vi "PICRv1.vi"() -> ()   [LabVIEW 2013]
uses:
  <vilib>/MakerHub/LINX/Public/Sensors/Accelerometer/MPU60X0/DeviceAddresses.ctl
  <vilib>/MakerHub/LINX/Public/Sensors/Accelerometer/MPU60X0/AccelFullScaleRanges.ctl
  <vilib>/MakerHub/LINX/Public/Sensors/Accelerometer/MPU60X0/GyroFullScaleRanges.ctl
  <vilib>/vision/Avi.llb/IMAQ AVI2 Refnum.ctl
  <vilib>/MakerHub/LINX/Public/Peripherals/Digital/Digital Write 1 Chan.vi
  <vilib>/MakerHub/LINX/Public/Peripherals/Digital/Digital Write N Chans.vi
  <vilib>/MakerHub/LINX/Private/Local IO/LinxDigitalWrite.vi
  <vilib>/MakerHub/LINX/Public/Utilities/Check Channel.vi
  <vilib>/MakerHub/LINX/Public/Utilities/Open Serial.vi
  <vilib>/MakerHub/LINX/Private/Utilties/Generate Error.vi
  <vilib>/picture/3D Picture Control/Object/Create Object (name).vi
  <vilib>/MakerHub/LINX/LMH-LINX.lvlib
  <vilib>/MakerHub/LINX/Public/Sensors/Accelerometer/MPU60X0/MPU60X0.lvlib
  <vilib>/picture/3D Picture Control/NI_3D Picture Control.lvlib
  <vilib>/vision/driver/NI_Vision_Acquisition_Software.lvlib
panel:
  out "Pressure":dbl
  in  "Stop":bool
  out "Image":T1(plugin-control)
  in  "Record":bool
  in  "AVI File Path":path=path "C:/Users/Deyaa/Desktop/op1.avi"
  in  "Motors":bool
  in  "Brush":bool
  in  "Stop/Start":bool
  out "Acceleration":T2(graph)
  in  "stop":bool
  out "Start/ Stop":bool
  out "Brush":bool
  out "Motors":bool
  in  "Slide":dbl(slide) scale=1.0..100.0
  out "3D Picture":refnum<vi>(3d-picture)
  out "Gyroscope":T2(graph)
  out "Temperature (°C)":dbl
  out "Acceleration  (dps)":T2
  in  "Stop":bool
  out "Gyro (g)":T2
  # "Gyroscope Simulation"
  # "Camera"
  # "IMU"
  # "Motion"
  # "Sinai University - Department Of Mechatronics\nGraduation Project 2017\nUnder Supervision Of Prof. Saber Abdrabbo\nDeyaa Muhammad"
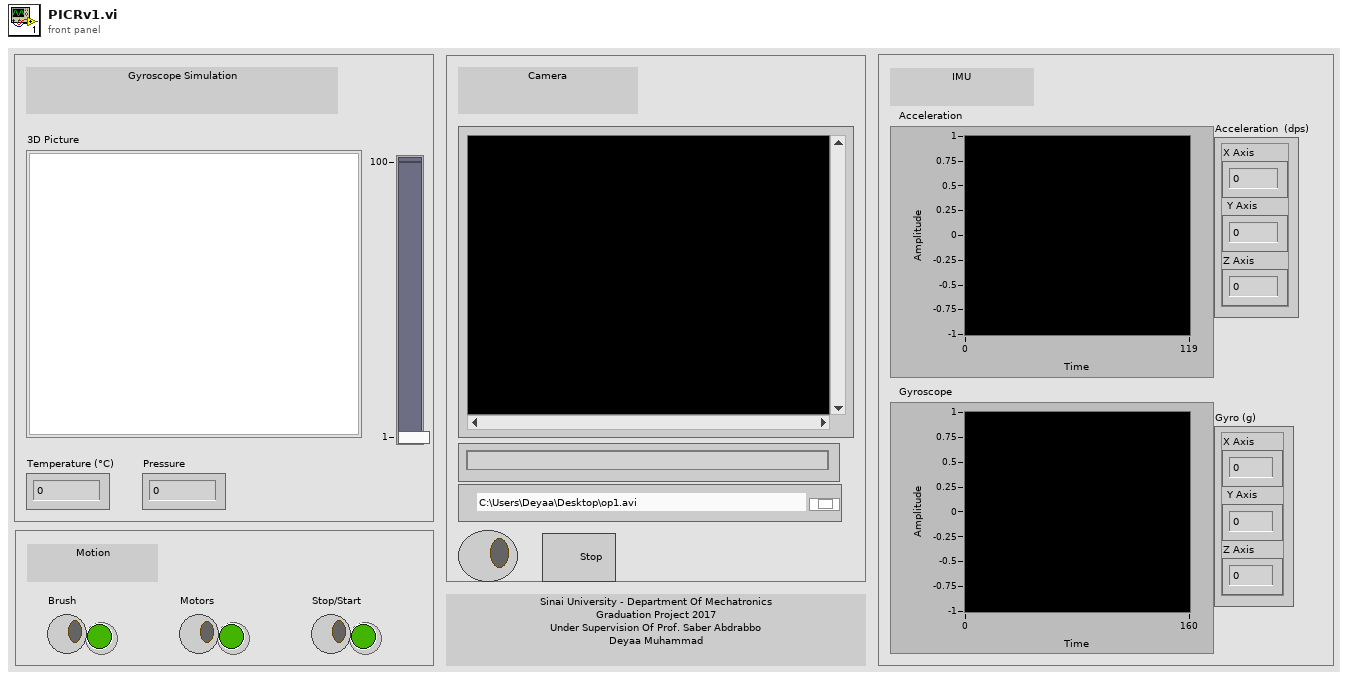
[diagram p1: front panel]
types:
  T1 = typedef "IMAQ Image.ctl" = refnum<image>
  T2 = cluster{"X Axis":i16, "Y Axis":i16, "Z Axis":i16}
  T3 = typedef "Image Type" = u32
  T4 = typedef "LMH-LINX.lvlib/MPU60X0.lvlib/GyroFullScaleRanges.ctl" = enum8{"±250 °/s", "±500 °/s", "±1000 °/s", "±2000 °/s"}
  T5 = typedef "LMH-LINX.lvlib/MPU60X0.lvlib/AccelFullScaleRanges.ctl" = enum16{"±2g", "±4g", "±8g", "±16g"}
  T6 = typedef "LMH-LINX.lvlib/MPU60X0.lvlib/DeviceAddresses.ctl" = enum16{"0x68", "0x69"}
  T7 = typedef "LMH-LINX.lvlib/LINX Ref.ctl" = cluster{"IO":T8, "Interface":T9, "LINX Device Config":T10}
  T8 = typedef "LMH-LINX.lvlib/Platform.ctl" = enum16{"Remote", "Local"}
  T9 = typedef "LMH-LINX.lvlib/Interface.ctl" = enum16{"Serial", "TCP"}
  T10 = typedef "LMH-LINX.lvlib/Device.lvlib/LINX Device Config.ctl" = cluster{"Interface":T9, "COM Port":refnum<visa-resource-name>, "TCP Configuration":T11, "Device Family":u8, "Device ID":u8, "Device Name":string, "TCP Ref":refnum<k5>, "Channels":T12}
  T11 = typedef "LMH-LINX.lvlib/Device.lvlib/TCP Config.ctl" = cluster{"IP Address":string, "Port":u16}
  T12 = typedef "LMH-LINX.lvlib/Channels.ctl" = cluster{"DI":u8[], "DO":u8[], "AI":u8[], "AO":u8[], "PWM":u8[], "QE":u8[], "UART":u8[], "I2C 2":u8[], "SPI":u8[], "CAN":u8[], "Servo":u8[], "AI Ref (V)":dbl, "AI Resolution (Bits)":u8, "AO Ref (V)":dbl, "AO Resolution (Bits)":u8}
  T13 = typedef "IMAQdx.ctl" = refnum<k21>
  T14 = typedef "IMAQ AVI2 Refnum.ctl" = refnum<k20>
  T15 = cluster{"Red":sgl, "Green":sgl, "Blue":sgl, "Alpha":sgl}
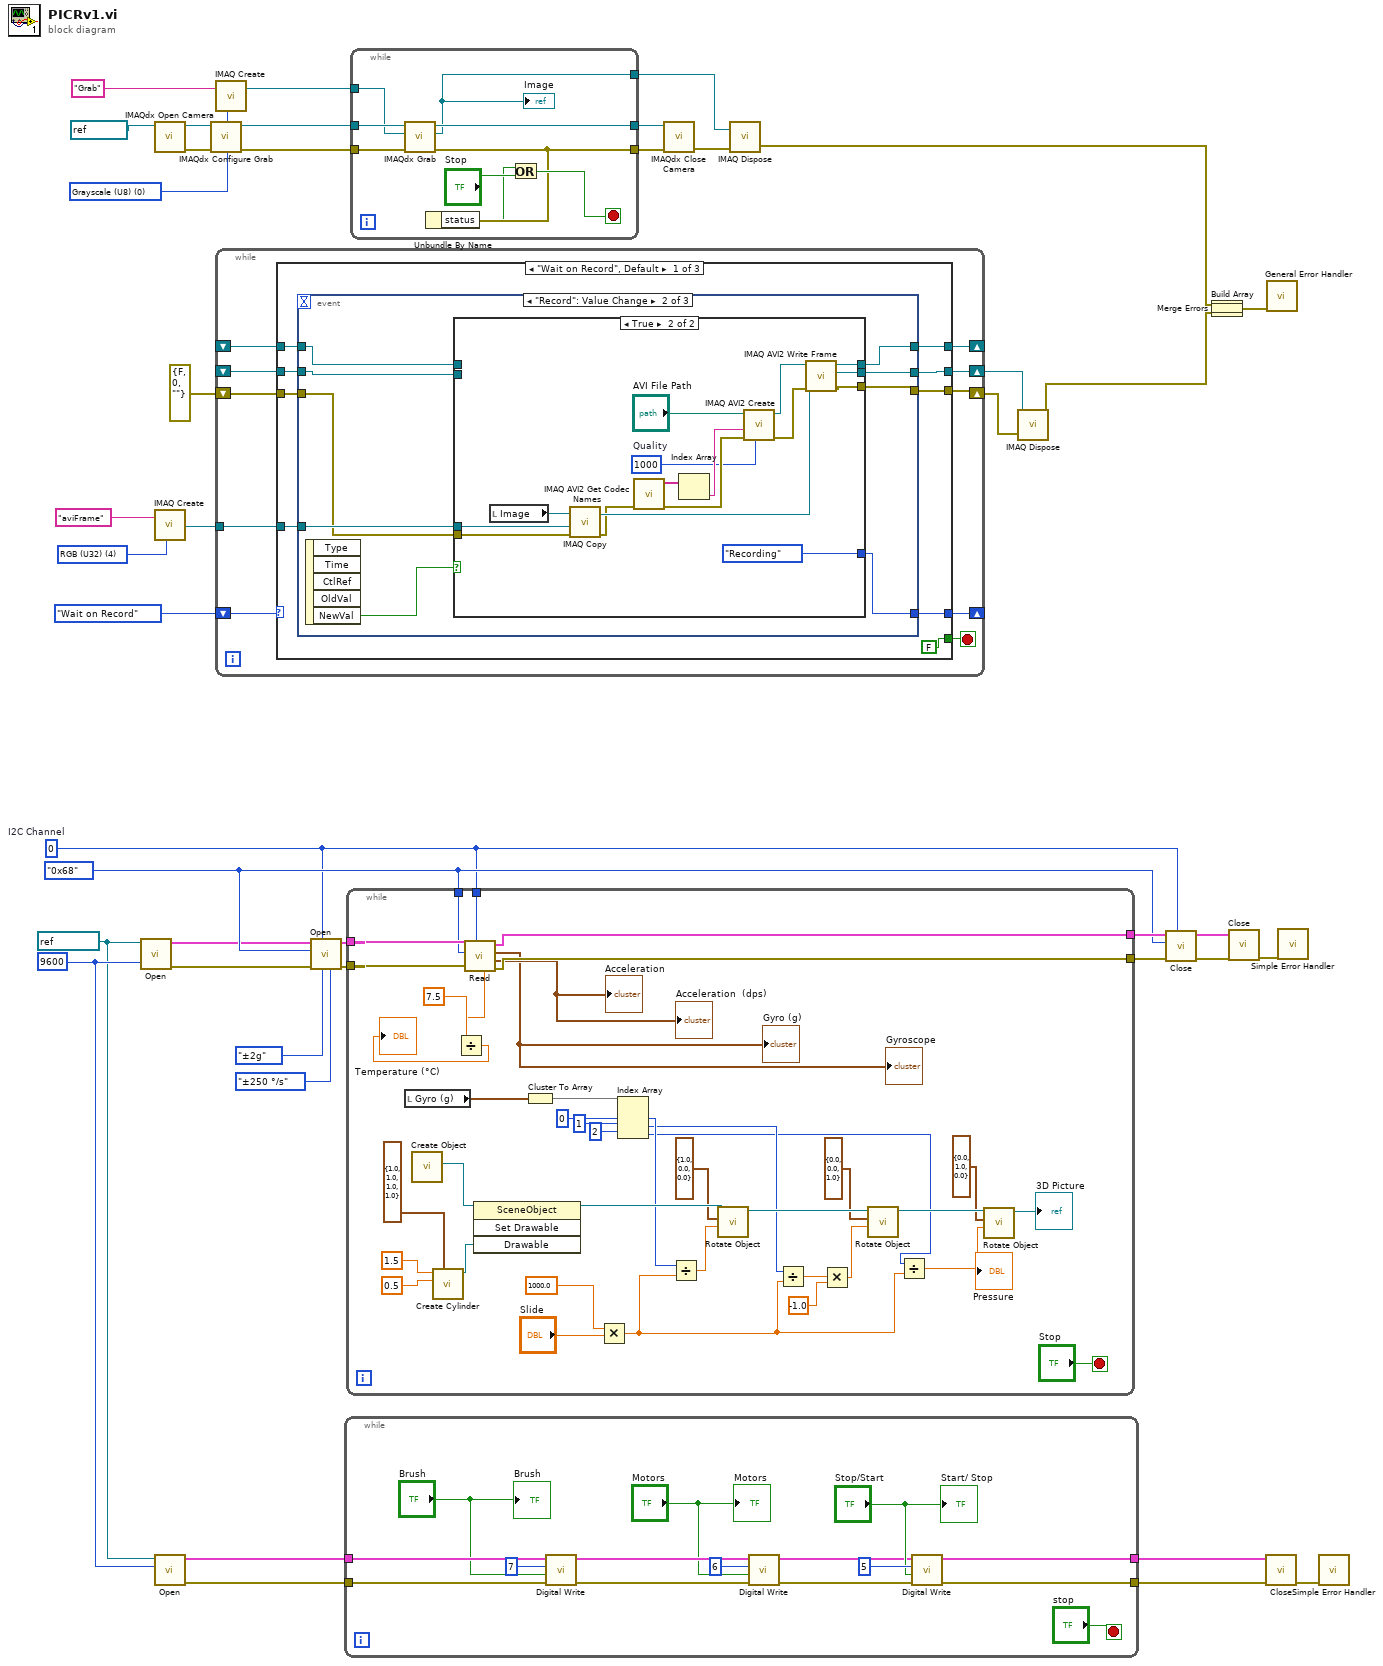
[diagram p0: block diagram]
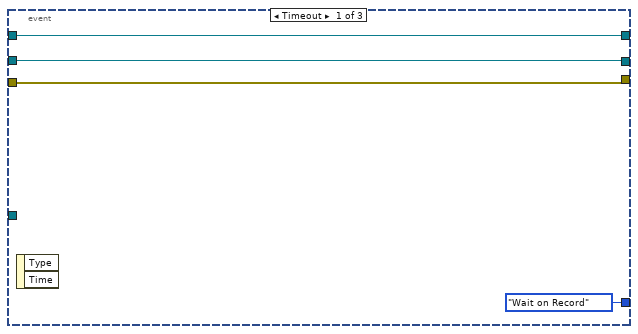
[diagram p2: hidden frame]
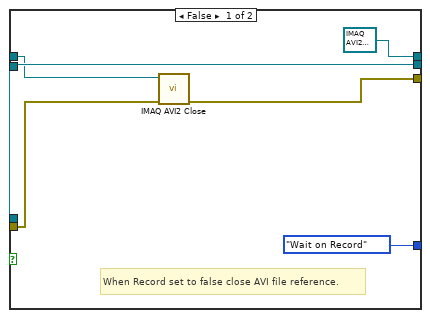
[diagram p3: hidden frame]
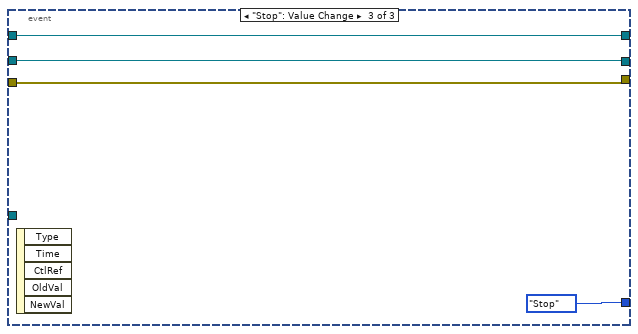
[diagram p4: hidden frame]
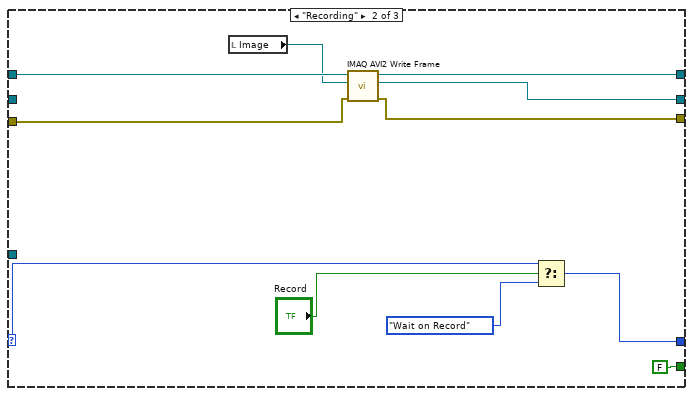
[diagram p5: hidden frame]
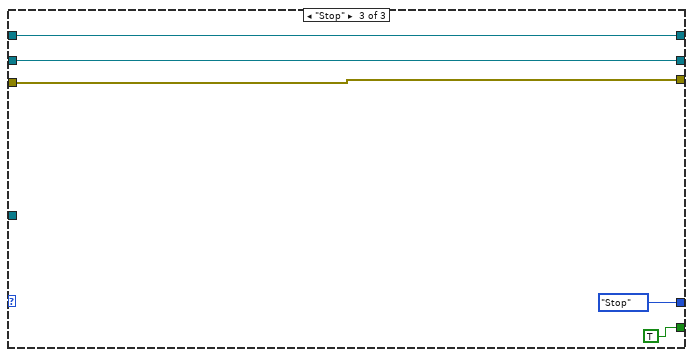
[diagram p6: hidden frame]
diagram:
  w6 = T3 0 items=["Grayscale (U8)", "Grayscale (I16)", "Grayscale (SGL)", "Complex (CSG)", "RGB (U32)", "HSL (U32)", "RGB (U64)", "Grayscale (U16)"] ("Image Type")
  w22 = T3 4 items=["Grayscale (U8)", "Grayscale (I16)", "Grayscale (SGL)", "Complex (CSG)", "RGB (U32)", "HSL (U32)", "RGB (U64)", "Grayscale (U16)"] ("Image Type")
  w34 = u8 0  # I2C Channel
  w1 = refnum<visa-resource-name> "COM3" ("Serial Port")
  w3 = u32 9600 ("Baud Rate Override")
  w38 = DeviceAddresses."0x68" ("I2C Slave Address")
  n1 = call-poly <vilib>:"Open.vi"("Baud Rate Override"=w3, "Serial Port"=w1) -> ("Error Out"=w32:errorcluster, "LINX Resource"=w33:T7)  [unwired: 7 in, 1 out]
  n2 = call <vilib>:"IMAQdx Open Camera.vi"("Session In"=refnum<k21> "cam1" ("Camera Name")) -> ("error out"=w13:errorcluster, "Session Out"=w12:T13)  [unwired: 2 in, 7 out]
  n3 = call "IMAQ Create"("Image Name"="aviFrame", "Image Type"=w22) -> ("New Image"=w25:T1)  [unwired: 3 in, 1 out]
  n4 = call-poly <vilib>:"Open.vi"("Baud Rate Override"=w3, "Serial Port"=w1) -> ("Error Out"=w29:errorcluster, "LINX Resource"=w30:T7)  [unwired: 7 in, 1 out]
  n5 = call <vilib>:"IMAQdx Configure Grab.vi"("error in"=w13, "Session In"=w12) -> ("error out"=w16:errorcluster, "Session Out"=w17:T13)  [unwired: 8 out]
  n6 = call "IMAQ Create"("Image Name"="Grab", "Image Type"=w6) -> ("New Image"=w18:T1)  [unwired: 2 in, 2 out]
  n7 = while {
    tunnel: w25 -> [w53]
    shift-right: [w49] -> _
    shift-left: enum16{"Wait on Record", "Recording", "Stop"}."Wait on Record" -> [w50]
    shift-right: [w48] -> _
    shift-left: _ -> [w47]
    shift-right: [w51] -> w23
    shift-left: errorcluster {"status"=FALSE, "code"=0, "source"=""} ("error out") -> [w46]
    shift-right: [w52] -> w24
    shift-left: _ -> [w44]
    stop <- w45 stop-if-true
    n8 = case shown="\"Wait on Record\", Default" w50 {
      selector: w50 -> [_ w102 _]
      tunnel: w53 -> [w62 _ _]
      tunnel: [w61 w105 w113] -> w52
      tunnel: [w60 w108 w115] -> w51
      tunnel: [w59 w107 enum16{"Wait on Record", "Recording", "Stop"}."Stop"] -> w49
      tunnel: [w58 w111 w116] -> w48
      tunnel: w47 -> [w57 w112 w116]
      tunnel: w46 -> [w56 w109 w115]
      tunnel: [FALSE FALSE TRUE] -> w45
      tunnel: w44 -> [w54 _ w113]
      frame "Wait on Record", Default {
        n9 = event shown="[1] \"Record\": Value Change" {
          selector: _ -> [_ _ _]
          dyn-events: _ -> [_ _ _]
          timeout: _ -> [_ _ _]
          tunnel: w62 -> [_ w75 _]
          tunnel: [w65 w74 w99] -> w61
          tunnel: [w66 w73 w98] -> w60
          tunnel: [enum16{"Wait on Record", "Recording", "Stop"}."Wait on Record" w67 enum16{"Wait on Record", "Recording", "Stop"}."Stop"] -> w59
          tunnel: [w64 w72 w100] -> w58
          tunnel: w57 -> [w64 w70 w100]
          tunnel: w56 -> [w66 w71 w98]
          tunnel: w54 -> [w65 w69 w99]
          event Timeout {
            n10 = event-data() -> ()  [unwired: 1 in, 2 out]
          }
          event "Record": Value Change {
            n11 = event-data() -> ("NewVal"=w68:bool)  [unwired: 1 in, 4 out]
            n12 = case shown="True" w68 {
              tunnel: w75 -> [w81 w97]
              tunnel: [w81 w90] -> w74
              tunnel: [w77 w89] -> w73
              tunnel: [T14 refnum ("AVI Refnum (duplicate)") w86] -> w72
              tunnel: w71 -> [w78 w83]
              tunnel: w70 -> [w79 _]
              tunnel: w69 -> [_ _]
              tunnel: [enum16{"Wait on Record", "Recording", "Stop"}."Wait on Record" enum16{"Wait on Record", "Recording", "Stop"}."Recording"] -> w67
              frame False {
                # "When Record set to false close AVI file reference."
                n13 = call "IMAQ AVI2 Close"("error in (no error)"=w78, "AVI Refnum"=w79) -> ("error out"=w77:errorcluster)  [unwired: 9 in]
              }
              frame True {
                w93 = 1000  # Quality
                n14 = local read "Image"() -> (w96:T1)
                n15 = call "IMAQ Copy"("error in (no error)"=w83, "Image Dst"=w97, "Image Src"=w96) -> ("error out"=w84:errorcluster, "Image Dst Out"=w88:T1)  [unwired: 3 in]
                n16 = call "IMAQ AVI2 Get Codec Names"("error in (no error)"=w84) -> ("error out"=w95:errorcluster, "Codec Names"=w92:string[])  [unwired: 9 in]
                n17 = Index Array(array=w92) -> (element=w94:string)  [unwired: 1 in]
                n18 = call "IMAQ AVI2 Create"("Quality"=w93, "error in (no error)"=w95, "Codec"=w94, "AVI Path"="AVI File Path") -> ("error out"=w85:errorcluster, "AVI Refnum"=w87:T14)  [unwired: 6 in]
                n19 = call "IMAQ AVI2 Write Frame"("error in (no error)"=w85, "Image"=w88, "AVI Refnum"=w87) -> ("error out"=w89:errorcluster, "Image Out (duplicate)"=w90:T1, "AVI Refnum (duplicate)"=w86:T14)  [unwired: 6 in]
              }
            }
          }
          event "Stop": Value Change {
            n20 = event-data() -> ()  [unwired: 1 in, 5 out]
          }
        }
      }
      frame "Recording" {
        n21 = local read "Image"() -> (w110:T1)
        n22 = call "IMAQ AVI2 Write Frame"("error in (no error)"=w109, "Image"=w110, "AVI Refnum"=w112) -> ("error out"=w108:errorcluster, "Image Out (duplicate)"=w105:T1, "AVI Refnum (duplicate)"=w111:T14)  [unwired: 6 in]
        n23 = Select(t=w102, s="Record", f=enum16{"Wait on Record", "Recording", "Stop"}."Wait on Record") -> (s? t:f=w107:enum16{"Wait on Record", "Recording", "Stop"})
      }
      frame "Stop" {
      }
    }
  }
  n24 = call <vilib>:"Open.vi"("Gyro Full Scale Range"=GyroFullScaleRanges."±250 °/s", "Accel Full Scale Range"=AccelFullScaleRanges."±2g", "I2C Channel"=w34, "Error In"=w32, "I2C Slave Address"=w38, "LINX Resource"=w33) -> ("Error Out"=w42:errorcluster, "LINX Resource"=w43:T7)  [unwired: 4 in]
  n25 = while {
    tunnel: w30 -> [w121]
    tunnel: w29 -> [w130]
    tunnel: [w129] -> w2
    tunnel: [w128] -> w28
    stop <- "stop" stop-if-true
    n26 = call-poly <vilib>:"Digital Write.vi"("Error In"=w130, "Output Value"="Brush", "DO Channel"=u8 7, "LINX Resource"=w121) -> ("Error Out"=w132:errorcluster, "LINX Resource"=w122:T7)  [unwired: 6 in]
    n27 = call-poly <vilib>:"Digital Write.vi"("Error In"=w132, "Output Value"="Motors", "DO Channel"=u8 6, "LINX Resource"=w122) -> ("Error Out"=w131:errorcluster, "LINX Resource"=w120:T7)  [unwired: 6 in]
    n28 = call-poly <vilib>:"Digital Write.vi"("Error In"=w131, "Output Value"="Stop/Start", "DO Channel"=u8 5, "LINX Resource"=w120) -> ("Error Out"=w128:errorcluster, "LINX Resource"=w129:T7)  [unwired: 6 in]
    "Motors" <- "Motors"
    "Brush" <- "Brush"
    "Start/ Stop" <- "Stop/Start"
  }
  n29 = while {
    tunnel: w43 -> [w172]
    tunnel: w42 -> [w171]
    tunnel: [w170] -> w41
    tunnel: [w169] -> w40
    tunnel: w38 -> [w167]
    tunnel: w34 -> [w166]
    stop <- "Stop" stop-if-true
    n30 = local read "Gyro (g)"() -> (w160:T2)
    n31 = call-poly <vilib>:"Create Object.vi"() -> ("Scene:New Object"=w155:refnum<vi>)  [unwired: 10 in, 1 out]
    n32 = call <vilib>:"Create Cylinder.vi"("Color"=T15 {"Red"=1.0, "Green"=1.0, "Blue"=1.0, "Alpha"=1.0}, "Radius"=sgl 0.5 ("Length Y"), "Height"=sgl 1.5 ("Length X")) -> ("New Cylinder Refnum"=w159:refnum<vi>)  [unwired: 7 in, 1 out]
    n33 = call <vilib>:"Read.vi"("I2C Channel"=w166, "Error In"=w171, "I2C Slave Address"=w167, "LINX Resource"=w172) -> ("Error Out"=w169:errorcluster, "Gyro  Data (dps)"=→"Acceleration  (dps)" →"Acceleration":T2, "Acceleration Data (g)"=→"Gyro (g)" →"Gyroscope":T2, "LINX Resource"=w170:T7, "Temperature (°C)"=w143:dbl)  [unwired: 3 in]
    n34 = Divide(x=w143, y=7.5) -> (x/y=→"Temperature (°C)":dbl)
    n35 = invoke class="SceneObject" method="Set Drawable"(reference=w155, "Drawable"=w159) -> (reference out=w164:refnum<vi>)  [unwired: 2 in, 3 out]
    n36 = Cluster To Array(cluster=w160) -> (array=w147:i16[])
    n37 = Multiply(x=1000.0, y="Slide") -> (x*y=w133:dbl)
    n38 = Index Array(array=w147, index #1=0 ("index"), index #2=1 ("index"), index #3=2 ("index")) -> (element #1=w154:i16, element #2=w135:i16, element #3=w134:i16)
    n39 = Divide(x=w154, y=w133) -> (x/y=w153:dbl)
    n40 = call <vilib>:"Rotate Object.vi"("Angle"=w153, "Axis"=cluster{"X":sgl, "Y":sgl, "Z":sgl} {"X"=1.0, "Y"=0.0, "Z"=0.0}, "Scene.Object In"=w164) -> ("Scene.Object Out"=w165:refnum<vi>)  [unwired: 7 in, 1 out]
    n41 = Divide(x=w135, y=w133) -> (x/y=w152:dbl)
    n42 = Multiply(x=w152, y=-1.0) -> (x*y=w150:dbl)
    n43 = call <vilib>:"Rotate Object.vi"("Angle"=w150, "Axis"=cluster{"X":sgl, "Y":sgl, "Z":sgl} {"X"=0.0, "Y"=0.0, "Z"=1.0}, "Scene.Object In"=w165) -> ("Scene.Object Out"=w149:refnum<vi>)  [unwired: 7 in, 1 out]
    n44 = Divide(x=w134, y=w133) -> (x/y=w139:dbl)
    n45 = call <vilib>:"Rotate Object.vi"("Angle"=w139, "Axis"=cluster{"X":sgl, "Y":sgl, "Z":sgl} {"X"=0.0, "Y"=1.0, "Z"=0.0}, "Scene.Object In"=w149) -> ("Scene.Object Out"=→"3D Picture":refnum<vi>)  [unwired: 7 in, 1 out]
  }
  n46 = while {
    tunnel: [w176] -> w15
    tunnel: w16 -> [w178]
    tunnel: w17 -> [w179]
    tunnel: [w175] -> w14
    tunnel: w18 -> [w177]
    tunnel: [w174] -> w11
    stop <- w181 stop-if-true
    n47 = call <vilib>:"IMAQdx Grab.vi"("error in"=w178, "Image In"=w177, "Session In"=w179) -> ("error out"=w175:errorcluster, "Image Out"=w174:T1, "Session Out"=w176:T13)  [unwired: 1 in, 5 out]
    "Image" <- w174
    n48 = Unbundle By Name(w175) -> ("status"=w173:bool)
    n49 = Or(x=w173, y="Stop") -> (x .or. y?=w181:bool)
  }
  n50 = call <vilib>:"IMAQdx Close Camera.vi"("error in"=w14, "Session In"=w15) -> ("error out"=w10:errorcluster)  [unwired: 9 out]
  n51 = call "IMAQ Dispose"("Image"=w11, "error in (no error)"=w10) -> ("error out"=w8:errorcluster)  [unwired: 4 in]
  n52 = call "IMAQ Dispose"("Image"=w24, "error in (no error)"=w23) -> ("error out"=w7:errorcluster)  [unwired: 1 in, 3 out]
  n53 = call <vilib>:"Close.vi"("I2C Channel (0)"=w34, "Error In"=w40, "I2C Slave Address (0)"=w38, "LINX Resource"=w41) -> ("Error Out"=w39:errorcluster, "LINX Resource"=w31:T7)  [unwired: 6 in]
  n54 = Build Array(w8, w7) -> (w5:errorcluster[])
  n55 = Merge Errors(w5) -> (w20:errorcluster)
  n56 = call <vilib>:"Close.vi"("Error In"=w39, "LINX Resource"=w31) -> ("Error Out"=w35:errorcluster)  [unwired: 9 in]
  n57 = call <vilib>:"Close.vi"("Error In"=w28, "LINX Resource"=w2) -> ("Error Out"=w27:errorcluster)  [unwired: 9 in]
  n58 = call <vilib>:"General Error Handler.vi"("error in (no error)"=w20) -> ()  [unwired: 1 in, 14 out]
  n59 = call <vilib>:"Simple Error Handler.vi"("error in (no error)"=w35) -> ()  [unwired: 4 in, 5 out]
  n60 = call <vilib>:"Simple Error Handler.vi"("error in (no error)"=w27) -> ()  [unwired: 4 in, 5 out]
